vi "TDMS Advanced Prefetched Asynchronous Read.vi"() -> ()   [LabVIEW 2023]
doc: "This example demonstrates how to read data asynchronously from a .tdms file using the Advanced TDMS VIs and functions. Users can specify a number of available buffers to read and stop the asynchronous reads and then read all the available data."
panel:
  out "Waveform Graph":u32[](graph)
  # "Overview: Demonstrates the use of the Advanced TDMS functions to read prefetched data from a .tdms file asynchronously.\nInstructions:\n1. Make sure you have already run TDMS Advanced Asynchronous Write.vi.\n2. Run this VI.\n3. Delete the TDMS file (located at [LabVIEW Data]\\Example TDMS Advanced Asynchronous Write.tdms) when you are done."
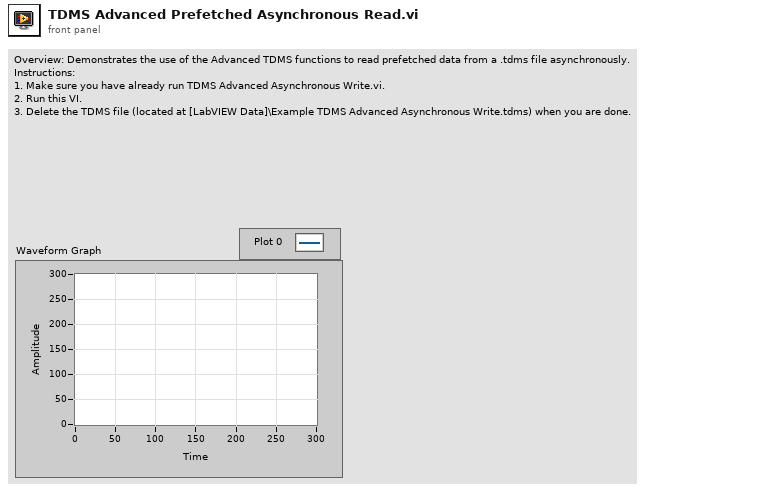
[diagram p1: front panel]
types:
  T1 = enum16{"open", "open or create", "create or replace", "create", "open (read-only)"}
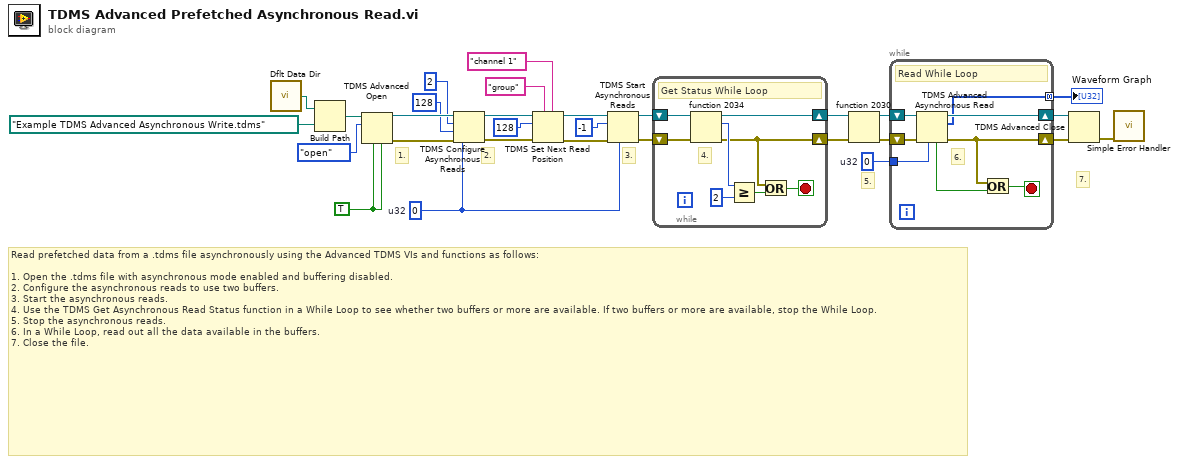
[diagram p0: block diagram]
diagram:
  w3 = u32 0  # u32
  w2 = u32 0  # u32
  w25 = TRUE ("enable asynchronous? (T)")
  # "5."
  # "3."
  # "2."
  # "Read prefetched data from a .tdms file asynchronously using the Advanced TDMS VIs and functions as follows:\n\n1. Open the .tdms file with asynchronous mode enabled and buffering disabled.\n2. Configure the asynchronous reads to use two buffers.\n3. Start the asynchronous reads.\n4. Use the TDMS Get Asynchronous Read Status function in a While Loop to see whether two buffers or more are available. If two buffers or more are available, stop the While Loop.\n5. Stop the asynchronous reads.\n6. In a While Loop, read out all the data available in the buffers.\n7. Close the file."
  # "1."
  # "7."
  n1 = call <vilib>:"Dflt Data Dir.vi"() -> ("App:Default Data Directory"=w26:path)
  n2 = Build Path(base path=w26, name or relative path=path "Example TDMS Advanced Asynchronous Write.tdms") -> (appended path=w28:path)
  n3 = TDMS Advanced Open(4:w25, 6:w25, 10:T1."open" ("operation (0:open)"), 11:w28) -> (0:w23:errorcluster, 3:w24:refnum<k34>)  [unwired: 1 in, 1 out]
  n4 = TDMS Configure Asynchronous Reads(6:w2, 8:w23, 9:u32 128 ("buffer size"), 10:u32 2 ("number of buffers (4)"), 11:w24) -> (0:w18:errorcluster, 3:w17:refnum<k34>)  [unwired: 1 in]
  n5 = TDMS Set Next Read Position(5:"channel 1" ("channel name in"), 7:"group" ("group name in"), 8:w18, 10:i64 128 ("offset (0)"), 11:w17) -> (0:w14:errorcluster, 3:w13:refnum<k34>)  [unwired: 1 in]
  n6 = TDMS Start Asynchronous Reads(6:w2, 8:w14, 10:i64 -1 ("total count (-1)"), 11:w13) -> (0:w19:errorcluster, 3:w20:refnum<k34>)
  n7 = while {
    shift-right: [w37] -> w11
    shift-left: w20 -> [w36]
    shift-right: [w30] -> w12
    shift-left: w19 -> [w35]
    stop <- w32 stop-if-true
    # "4."
    # "Get Status While Loop"
    n8 = fn#2034(8:w35, 11:w36) -> (0:w30:errorcluster, 2:w34:u32, 3:w37:refnum<k34>)  [unwired: 1 out]
    n9 = Greater Or Equal?(x=w34, y=u32 2) -> (x >= y?=w33:bool)
    n10 = Or(x=w30, y=w33) -> (x .or. y?=w32:bool)
  }
  n11 = fn#2030(8:w12, 11:w11) -> (0:w7:errorcluster, 3:w8:refnum<k34>)
  n12 = while {
    shift-right: [w38] -> w10
    shift-left: w7 -> [w42]
    shift-right: [w45] -> w9
    shift-left: w8 -> [w43]
    tunnel: w3 -> [w44]
    tunnel: [w39] -> w1 mode=concatenating
    stop <- w40 stop-if-true
    # "6."
    # "Read While Loop"
    n13 = TDMS Advanced Asynchronous Read(6:w44, 8:w42, 11:w43) -> (0:w38:errorcluster, 2:w39:u32[], 3:w45:refnum<k34>, 4:w41:bool)
    n14 = Or(x=w38, y=w41) -> (x .or. y?=w40:bool)
  }
  "Waveform Graph" <- w1
  n15 = TDMS Advanced Close(8:w10, 11:w9) -> (0:w6:errorcluster)  [unwired: 2 in, 1 out]
  n16 = call <vilib>:"Simple Error Handler.vi"("error in (no error)"=w6) -> ()  [unwired: 4 in, 5 out]
